vi "Write Test Listbox.vi"(8 "Value":i32, 9 "Symbols":i32[](array[numeric]), 10 "Measurement Names":string[](array[string]), 11 "Test Framework in":refnum<class "Test Framework.lvclass">) -> (3 "Test Framework out":refnum<class "Test Framework.lvclass">)   [LabVIEW 2020, in "Test Framework.lvclass"]
uses:
  Test Framework.lvclass
  Test Framework.lvclass/Test Framework.ctl
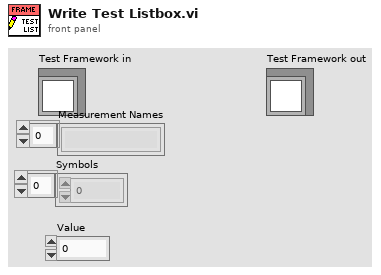
[diagram p1: front panel]
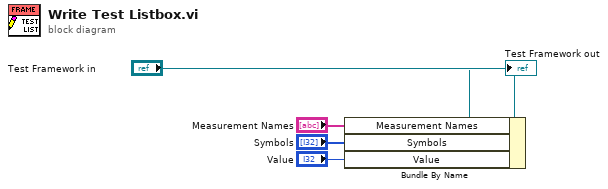
[diagram p0: block diagram]
diagram:
  n1 = Bundle By Name(cluster="Test Framework in", "Measurement Names"="Measurement Names", "Symbols"="Symbols", "Value"="Value") -> (→"Test Framework out":refnum<class "Test Framework.lvclass">)
